vi "3D Curve graph.vi"() -> (1 "3D graph out":refnum<k7>, 2 "Latitude out":dbl format="%.2f", 3 "Longitude out":dbl format="%.2f")   [LabVIEW 2013]
uses:
  <vilib>/Platform/NI_3dgraph.lvlib
panel:
  out "error out":errorcluster
  in  "3D Surface":refnum<k7>(container)
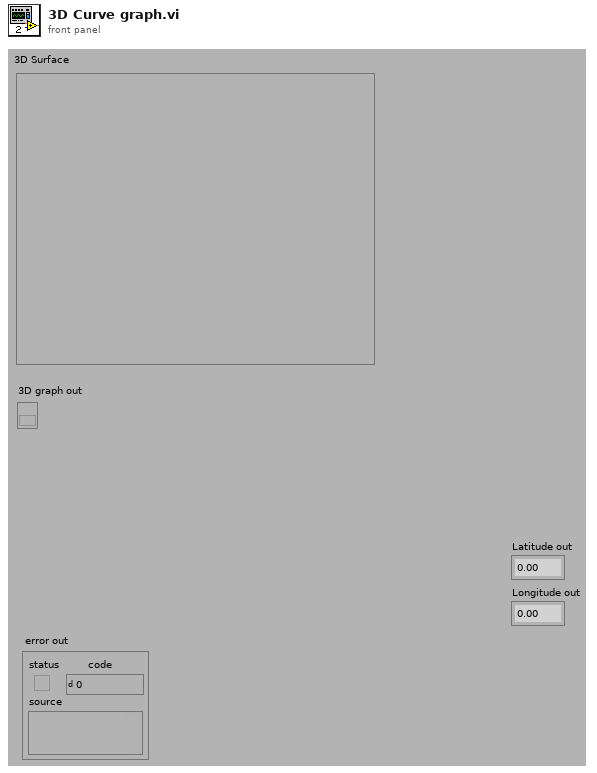
[diagram p1: front panel]
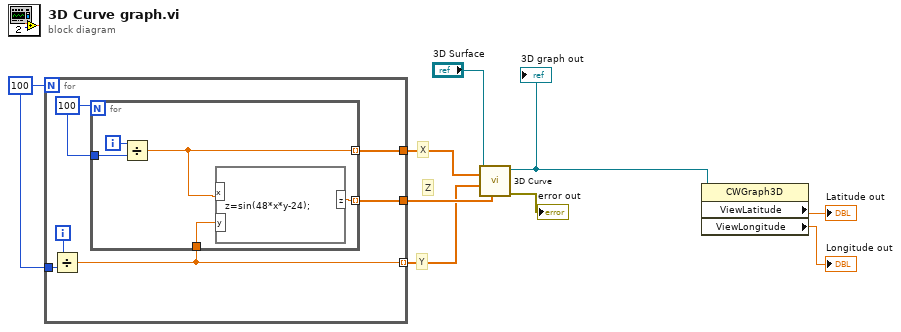
[diagram p0: block diagram]
diagram:
  w9 = 100
  # "Z"
  # "X"
  # "Y"
  n1 = for {
    N: w9 -> [_]
    tunnel: w9 -> [w13]
    tunnel: [w12] -> w1
    tunnel: [w11] -> w2 mode=indexing
    tunnel: [w10] -> w3
    i -> [w14]
    w15 = 100
    n2 = Divide(x=w14, y=w13) -> (x/y=w11:dbl)
    n3 = for {
      N: w15 -> [_]
      tunnel: w15 -> [w19]
      tunnel: [w18] -> w12 mode=indexing
      tunnel: w11 -> [w16]
      tunnel: [w17] -> w10 mode=indexing
      i -> [w20]
      n4 = Divide(x=w20, y=w19) -> (x/y=w18:dbl)
      n5 = formula code="z=sin(48*x*y-24);"("y"=w16, "x"=w18) -> ("z"=w17:dbl)
    }
  }
  n6 = call <vilib>:"3D Curve.vi"("z vector"=w3, "y vector"=w2, "x vector"=w1, "3D graph"="3D Surface") -> ("error out"=→"error out":errorcluster, "3D graph out"=w5:refnum<k7>)  [unwired: 1 in, 5 out]
  "3D graph out" <- w5
  n7 = property class="CWGraph3D"(reference=w5) -> ("ViewLatitude"=→"Latitude out":dbl, "ViewLongitude"=→"Longitude out":dbl)  [unwired: 1 in, 2 out]
